vi "Read ADC.vi"(8 "error in (no error)":errorcluster, 10 "canal":dbl, 11 "Arduino in":refnum<class "Arduino.lvclass">) -> (0 "error out":errorcluster, 3 "Arduino out":refnum<class "Arduino.lvclass">)   [LabVIEW 2019, in "Arduino.lvclass"]
uses:
  Arduino.lvclass
  Arduino.lvclass/Arduino.ctl
  9556c618-0d6e-4ad1-833e-7019577c3cef.vi
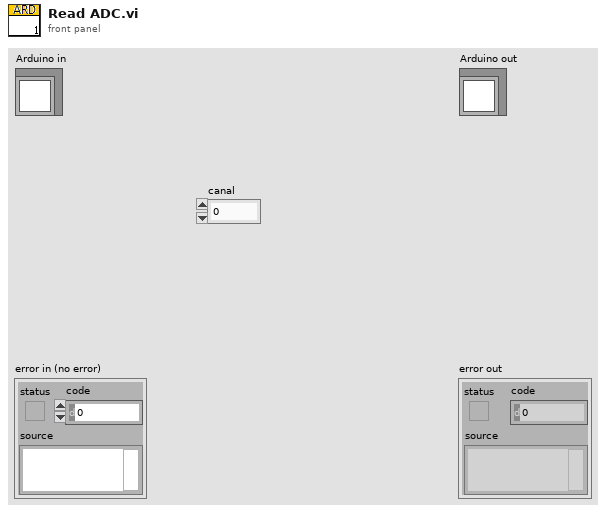
[diagram p1: front panel]
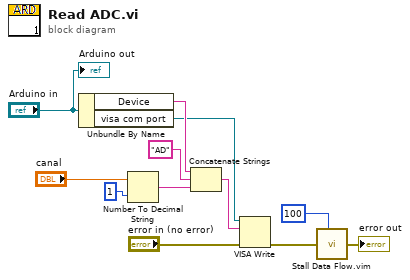
[diagram p0: block diagram]
diagram:
  n1 = Unbundle By Name("Arduino in") -> ("Device"=w9:string, "visa com port"=w5:refnum<visa-resource-name>)
  n2 = Number To Decimal String(number="canal", width (-)=i16 1) -> (decimal integer string=w7:string)
  n3 = Concatenate Strings(w9, "AD" ("string"), w7) -> (w6:string)
  n4 = VISA Write(VISA resource name=w5, write buffer=w6, error in (no error)="error in (no error)") -> (error out=w3:errorcluster)  [unwired: 2 out]
  n5 = call "Stall Data Flow.vim"("value in"=w3, "milliseconds to wait"=u32 100) -> ("value out"=→"error out":errorcluster)  [unwired: 1 out]
  "Arduino out" <- "Arduino in"
